vi "File_WriteLog.vi"(8 "error in (no error)":errorcluster, 9 "dt per loop":dbl, 10 "Loop Counter":i32, 11 "File in":refnum<class "File.lvclass">) -> (0 "error out":errorcluster, 3 "File out":refnum<class "File.lvclass">)   [LabVIEW 2023, in "File.lvclass"]
doc: "Is a top level VI which has all subsidiary channels log to file."
uses:
  File.lvclass
  File.lvclass/File.ctl
  Group/Group.lvclass
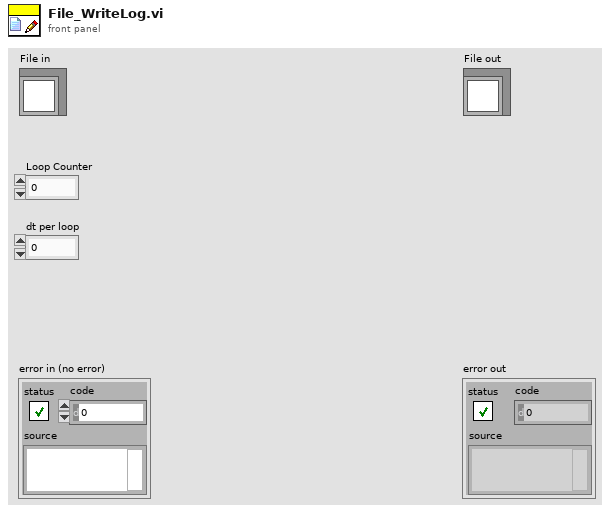
[diagram p1: front panel]
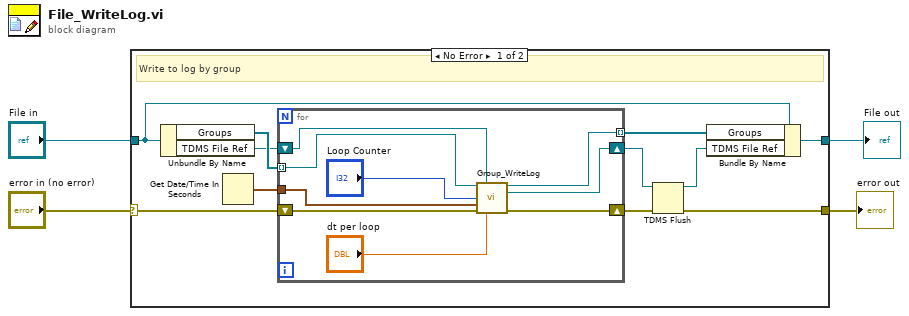
[diagram p0: block diagram]
diagram:
  n1 = case shown="No Error" "error in (no error)" {
    selector: "error in (no error)" -> [w8 w26]
    tunnel: [w9 w26] -> w3
    tunnel: [w12 w25] -> w1
    tunnel: "File in" -> [w13 w25]
    frame No Error {
      # "Write to log by group"
      n2 = Unbundle By Name(w13) -> ("Groups"=w15:refnum<class "Group.lvclass">[], "TDMS File Ref"=w7:refnum<k34>)
      n3 = Get Date/Time In Seconds() -> (seconds since 1Jan1904=w14:timestamp)
      n4 = for {
        tunnel: w15 -> [w24] mode=indexing
        tunnel: w14 -> [w19]
        shift-right: [w23] -> w10
        shift-left: w8 -> [w22]
        tunnel: [w18] -> w6 mode=indexing
        shift-right: [w17] -> w11
        shift-left: w7 -> [w16]
        n5 = call-dynamic "Group_WriteLog.vi"("Group in"=w24, "tdms file"=w16, "Loop Counter"="Loop Counter", "t0"=w19, "error in (no error)"=w22, "dt per loop"="dt per loop") -> ("Group out"=w18:refnum<class "Group.lvclass">, "tdms file out"=w17:refnum<k34>, "error out"=w23:errorcluster)  [unwired: 7 in]
      }
      n6 = TDMS Flush(4:w10, 7:w11) -> (0:w9:errorcluster, 3:w5:refnum<k34>)
      n7 = Bundle By Name(cluster=w13, "Groups"=w6, "TDMS File Ref"=w5) -> (w12:refnum<class "File.lvclass">)
    }
    frame Error {
    }
  }
  "error out" <- w3
  "File out" <- w1
